vi "L0 Asic Test.vi"() -> ()   [LabVIEW 2009]
uses:
  <vilib>/Utility/file.llb/Write To Spreadsheet File (string).vi
  <vilib>/Analysis/NI_AALBase.lvlib
panel:
  out "Channel":i32
  out "Delay Index":u16(ring) items=["0", "0.25ns", "0.5ns", "0.75ns", "1ns", "1.25ns", "1.5ns", "1.75ns", "2ns", "2.25ns", "2.5ns", "2.75ns", "3ns", "3.25ns", "3.5ns", "3.75ns", "4ns", "4.25ns", "4.5ns", "4.75ns", "5ns", "5.25ns", "5.5ns", "5.75ns", "2ns_b", "2.25ns_b", "2.5ns_b", "2.75ns_b", "3ns_b", "3.25ns_b", "3.5ns_b", "3.75ns_b", ""]
  in  "error in 1":errorcluster
  out "error 2 out":errorcluster
  out "VISA resource name out":refnum<visa-resource-name>="Oscilloscope"
  in  "Osc":refnum<visa-resource-name>="Oscilloscope"
  in  "Generator":refnum<visa-resource-name>="generadorpulsos"
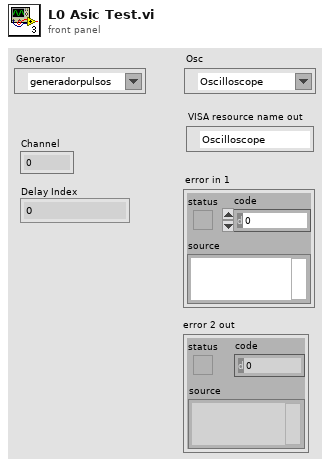
[diagram p1: front panel]
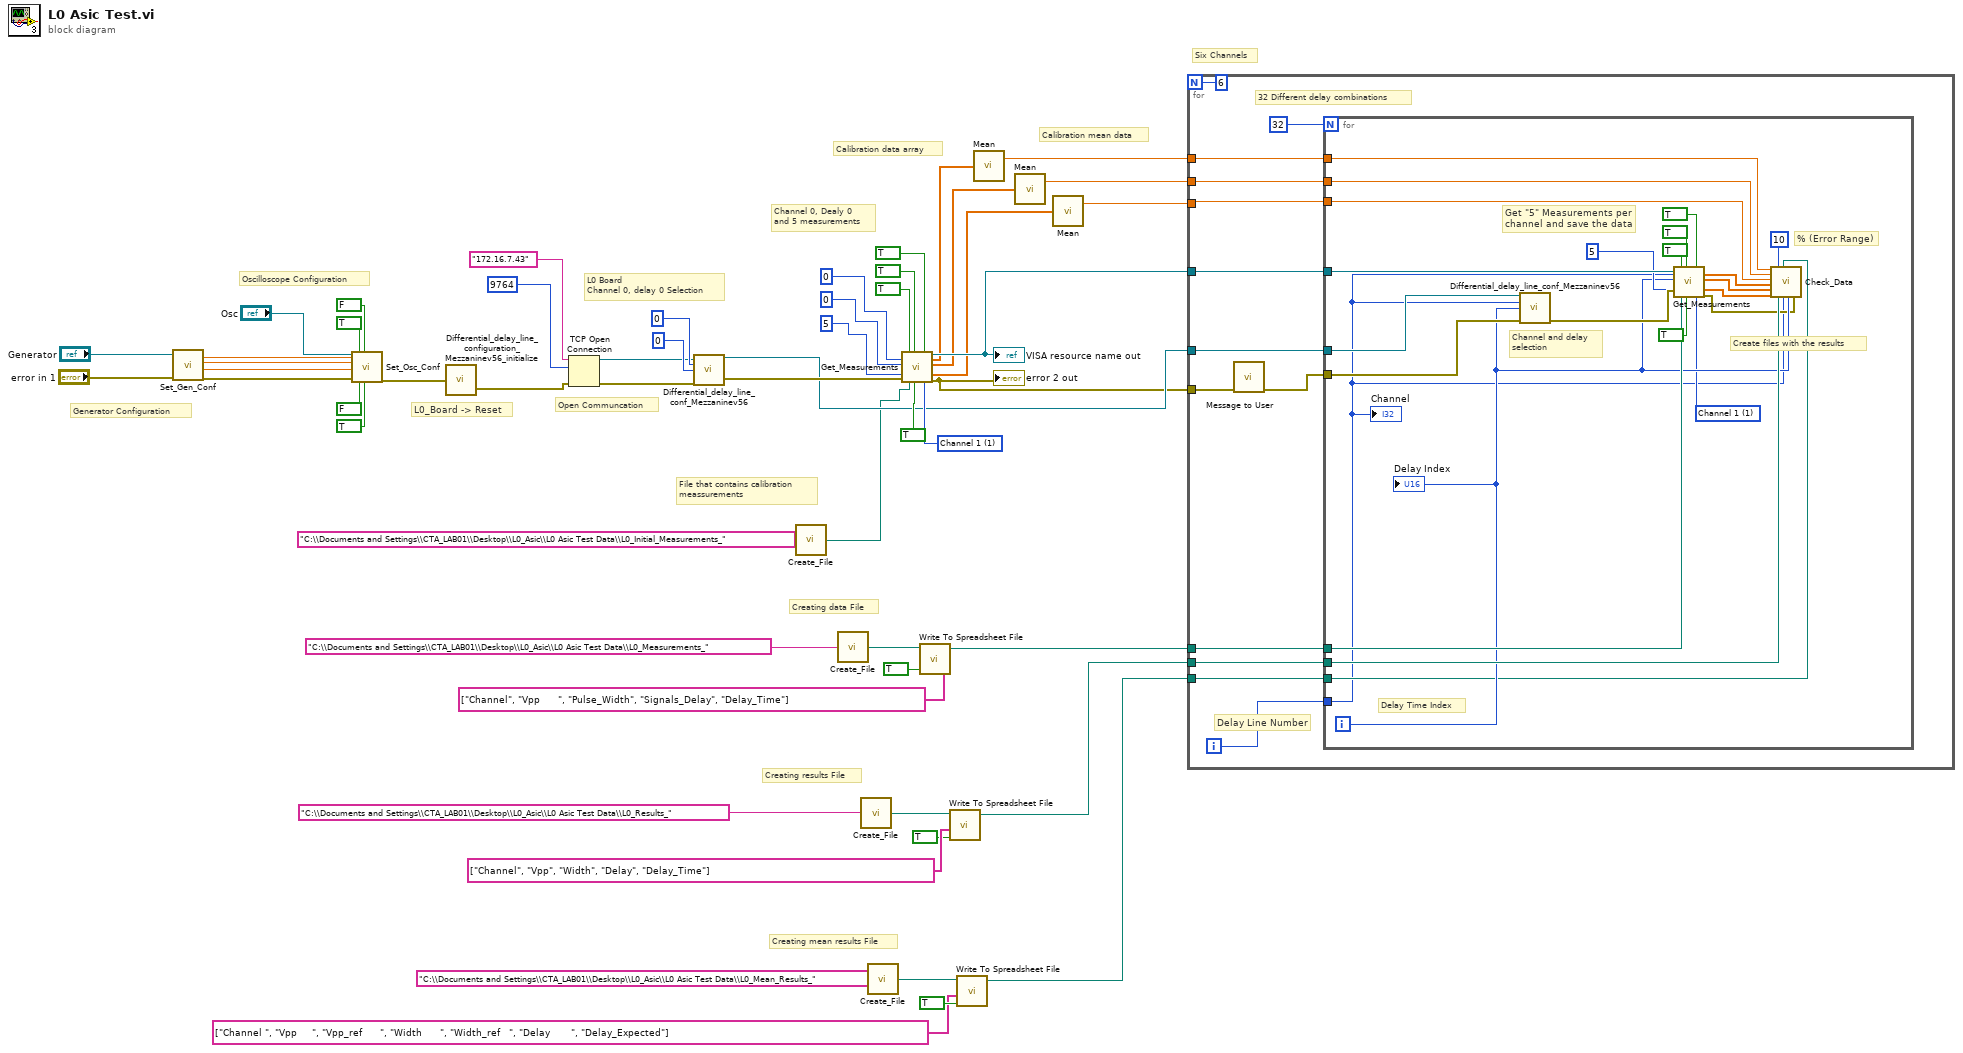
[diagram p0: block diagram]
diagram:
  w26 = 1 items=["Channel 1"=1, "Channel 2"=2, "Channel 3"=3, "Channel 4"=4, "Function 1"=5, "Function 2"=6, "Function 3"=7, "Function 4"=8, "Memory 1"=9, "Memory 2"=10, "Memory 3"=11, "Memory 4"=12] ("Channel")
  # "Creating mean results File"
  # "Calibration mean data"
  # "Calibration data array"
  # "File that contains calibration \nmeassurements"
  # "Open Communcation"
  # "Oscilloscope Configuration"
  # "Generator Configuration"
  # "L0 Board\nChannel 0, delay 0 Selection"
  # "Channel 0, Dealy 0\nand 5 measurements"
  # "Six Channels"
  # "L0_Board -> Reset"
  # "Creating results File"
  # "Creating data File"
  n1 = call "Set_Gen_Conf.vi"("AWG VISA"="Generator", "error in (no error)"="error in 1") -> ("Amplitude 1 OUT"=w48:dbl, "Pulse Width in seconds 1 OUT"=w47:dbl, "Trigger Level 1"=w46:dbl, "error out"=w44:errorcluster)  [unwired: 10 in, 4 out]
  n2 = call "Set_Osc_Conf.vi"("VISA resource name"="Osc", "Amplitude IN"=w48, "Trigger Level IN"=w46, "Pulse Width in seconds IN"=w47, "error in (no error)"=w44, "Channel 1"=TRUE, "Channel 3"=FALSE, "Channel 2"=FALSE, "Channel 4"=TRUE) -> ("error out"=w38:errorcluster)  [unwired: 9 in, 1 out]
  n3 = call "Differential_delay_line_configuration_Mezzaninev56_initialize.vi"("error in (no error)"=w38) -> ("error out 2"=w18:errorcluster)  [unwired: 1 in]
  n4 = TCP Open Connection(address="172.16.7.43", remote port or service name=u16 9764, error in (no error)=w18) -> (connection ID=w16:refnum<k5>, error out=w17:errorcluster)  [unwired: 2 in]
  n5 = call "Differential_delay_line_conf_Mezzaninev56.vi"("connection ID"=w16, "channel"=0, "Delay value"=u16 0, "error in (no error)"=w17) -> ("connection ID out"=w14:refnum<k5>, "error out 2"=w15:errorcluster)  [unwired: 4 in, 6 out]
  n6 = call "Create_File.vi"("String"="C:\\Documents and Settings\\CTA_LAB01\\Desktop\\L0_Asic\\L0 Asic Test Data\\L0_Initial_Measurements_") -> ("path"=w6:path)
  n7 = call "Create_File.vi"("String"="C:\\Documents and Settings\\CTA_LAB01\\Desktop\\L0_Asic\\L0 Asic Test Data\\L0_Measurements_") -> ("path"=w12:path)
  n8 = call "Create_File.vi"("String"="C:\\Documents and Settings\\CTA_LAB01\\Desktop\\L0_Asic\\L0 Asic Test Data\\L0_Results_") -> ("path"=w10:path)
  n9 = call "Create_File.vi"("String"="C:\\Documents and Settings\\CTA_LAB01\\Desktop\\L0_Asic\\L0 Asic Test Data\\L0_Mean_Results_") -> ("path"=w5:path)
  n10 = call "Get_Measurements.vi"("Delay_Index"=0, "Measurements per channel"=5, "Amplitude"=TRUE ("Delay"), "file path (dialog if empty)"=w6, "Width"=TRUE, "Write to a file?"=TRUE, "Delay_Line_Number"=0, "error in"=w15, "Delay"=TRUE ("Amplitude"), "Oscilloscope Channel"=w26) -> ("VISA resource name out"=w34:refnum<visa-resource-name>, "Vpp_Array"=w32:dbl[], "Width Array"=w30:dbl[], "Setup_Time_Array"=w29:dbl[], "error out"=w13:errorcluster)  [unwired: 5 in]
  "VISA resource name out" <- w34
  "error 2 out" <- w13
  n11 = call-poly <vilib>:"Write To Spreadsheet File.vi"("append to file? (new file:F)"=TRUE, "1D data"=string[] ["Channel", "Vpp      ", "Pulse_Width", "Signals_Delay", "Delay_Time"], "file path (dialog if empty)"=w12) -> ("new file path (Not A Path if cancelled)"=w40:path)  [unwired: 5 in]
  n12 = call-poly <vilib>:"Write To Spreadsheet File.vi"("append to file? (new file:F)"=TRUE, "1D data"=string[] ["Channel", "Vpp", "Width", "Delay", "Delay_Time"], "file path (dialog if empty)"=w10) -> ("new file path (Not A Path if cancelled)"=w39:path)  [unwired: 5 in]
  n13 = call-poly <vilib>:"Write To Spreadsheet File.vi"("append to file? (new file:F)"=TRUE, "1D data"=string[] ["Channel ", "Vpp     ", "Vpp_ref      ", "Width      ", "Width_ref   ", "Delay       ", "Delay_Expected"], "file path (dialog if empty)"=w5) -> ("new file path (Not A Path if cancelled)"=w2:path)  [unwired: 5 in]
  n14 = call <vilib>:"Mean.vi"("X"=w32) -> ("mean"=w33:dbl)  [unwired: 1 out]
  n15 = call <vilib>:"Mean.vi"("X"=w30) -> ("mean"=w31:dbl)  [unwired: 1 out]
  n16 = call <vilib>:"Mean.vi"("X"=w29) -> ("mean"=w28:dbl)  [unwired: 1 out]
  n17 = for {
    N: 6 -> [_]
    tunnel: w14 -> [w67]
    tunnel: w13 -> [w59]
    tunnel: w34 -> [w66]
    tunnel: w40 -> [w64]
    tunnel: w39 -> [w61]
    tunnel: w33 -> [w63]
    tunnel: w28 -> [w60]
    tunnel: w31 -> [w62]
    tunnel: w2 -> [w57]
    i -> [w56]
    # "Delay Line Number"
    # "32 Different delay combinations"
    n18 = call "Message to User"("error in (no error)"=w59) -> ("error out"=w58:errorcluster)  [unwired: 9 in, 1 out]
    n19 = for {
      N: 32 -> [_]
      tunnel: w67 -> [w90]
      tunnel: w58 -> [w89]
      tunnel: w56 -> [w68]
      tunnel: w66 -> [w88]
      tunnel: w64 -> [w85]
      tunnel: w63 -> [w84]
      tunnel: w62 -> [w83]
      tunnel: w60 -> [w76]
      tunnel: w61 -> [w78]
      tunnel: w57 -> [w69]
      i -> [w77]
      w70 = 1 items=["Channel 1"=1, "Channel 2"=2, "Channel 3"=3, "Channel 4"=4, "Function 1"=5, "Function 2"=6, "Function 3"=7, "Function 4"=8, "Memory 1"=9, "Memory 2"=10, "Memory 3"=11, "Memory 4"=12] ("Oscilloscope Channel")
      # "Create files with the results"
      # "Channel and delay\nselection"
      # "Delay Time Index"
      # "% (Error Range)"
      # "Get \"5\" Measurements per \nchannel and save the data"
      n20 = call "Differential_delay_line_conf_Mezzaninev56.vi"("connection ID"=w90, "channel"=w68, "Delay value"=w77, "error in (no error)"=w89) -> ("error out 2"=w87:errorcluster)  [unwired: 4 in, 7 out]
      n21 = call "Get_Measurements.vi"("VISA resource name"=w88, "Delay_Index"=w77, "Measurements per channel"=5, "Amplitude"=TRUE ("Delay"), "file path (dialog if empty)"=w85, "Width"=TRUE, "Write to a file?"=TRUE, "Delay_Line_Number"=w68, "error in"=w87, "Delay"=TRUE ("Amplitude"), "Oscilloscope Channel"=w70) -> ("Vpp_Array"=w82:dbl[], "Width Array"=w81:dbl[], "Setup_Time_Array"=w80:dbl[], "error out"=w75:errorcluster)  [unwired: 4 in, 1 out]
      n22 = call "Check_Data.vi"("Vpp_0"=w84, "Width_0"=w83, "Setup_Time_0"=w76, "Vpp_Array"=w82, "Width Array"=w81, "Setup_Time_Array"=w80, "Percentage_Range"=10, "file path (dialog if empty)"=w78, "file path (dialog if empty) 2"=w69, "Delay Line Number"=w68, "Delay Index"=w77, "error in 1"=w75) -> ()  [unwired: 7 in, 1 out]
      "Delay Index" <- w77
      "Channel" <- w68
    }
  }
